vi "PhotonPoseEstimator_closestToReferencePoseStrategy.vi"(9 "ReferencePose":T2={"Translation3d"={"X"=0.0, "Y"=0.0, "Z"=0.0}, "Rotation3d"={"Q_quaternion"={"R"=1.0, "V"=[0.0, 0.0, 0.0]}}} {"Translation3d"."Z" format="%14.3f"; "Translation3d"."Y" format="%14.3f"; "Translation3d"."X" format="%14.3f"}, 10 "CameraResult":T11, 11 "PhotonPoseEstimator_REF":T1) -> (1 "Pos Found":bool, 3 "PhotonEstimatedRobotPose":T6={"EstimatedPose"={"Translation3d"={"X"=0.0, "Y"=0.0, "Z"=0.0}, "Rotation3d"={"Q_quaternion"={"R"=1.0, "V"=[0.0, 0.0, 0.0]}}}, "TimeStamp_Seconds"=0.0, "targetsUsed"=[], "Strategy"=enum."LOWEST_AMBIGUITY"} {"targetsUsed"."AltCameraToTarget"."TRANSLATION3D"."Z" format="%14.3f"; "targetsUsed"."AltCameraToTarget"."TRANSLATION3D"."Y" format="%14.3f"; "targetsUsed"."AltCameraToTarget"."TRANSLATION3D"."X" format="%14.3f"; "targetsUsed"."BestCameraToTarget"."TRANSLATION3D"."Z" format="%14.3f"; "targetsUsed"."BestCameraToTarget"."TRANSLATION3D"."Y" format="%14.3f"; "targetsUsed"."BestCameraToTarget"."TRANSLATION3D"."X" format="%14.3f"; "EstimatedPose"."Translation3d"."Z" format="%14.3f"; "EstimatedPose"."Translation3d"."Y" format="%14.3f"; "EstimatedPose"."Translation3d"."X" format="%14.3f"})   [LabVIEW 2019, in "PhotonVisionLib.lvlib"]
doc: "This is an internal function. Use Update or Update_Pipeline instead of this function.\n\nDetermine the best target based on the closest to a set Reference position"
uses:
  PhotonVisionLib.lvlib
  <vilib>/Rock Robotics/WPI/ThirdParty/JAS_Junk/TrajLib/TypeDef/QUATERNION.ctl
  <vilib>/Rock Robotics/WPI/ThirdParty/JAS_Junk/TrajLib/Trajectory_Library.lvlib
  <vilib>/Rock Robotics/WPI/ThirdParty/JAS_Junk/TrajLib/TypeDef/ROTATION3D.ctl
  <vilib>/Rock Robotics/WPI/ThirdParty/JAS_Junk/TrajLib/TypeDef/TRANSLATION3D.ctl
  <vilib>/Rock Robotics/WPI/ThirdParty/JAS_Junk/TrajLib/TypeDef/POSE3D.ctl
  TypeDef/PhotonEstimatedRobotPoseType.ctl
  Enum/PhotonPoseStrategy_ENUM.ctl
  TypeDef/TargetCornerType.ctl
  <vilib>/Rock Robotics/WPI/ThirdParty/JAS_Junk/TrajLib/TypeDef/TRANSFORM3D.ctl
  TypeDef/PhotonTrackedTargetType.ctl
  TypeDef/PhotonPipelineResultType.ctl
  <vilib>/Rock Robotics/WPI/ThirdParty/JAS_Junk/TrajLib/TypeDef/AprilTag.ctl
  <vilib>/Rock Robotics/WPI/ThirdParty/JAS_Junk/TrajLib/Enum/AprilTagFieldLayoutOrignPosition_ENUM.ctl
  <vilib>/Rock Robotics/WPI/ThirdParty/JAS_Junk/TrajLib/TypeDef/AprilTagFieldLayout.ctl
  TypeDef/PhotonPoseEstimatorType.ctl
  TypeDef/PhotonPNPResultType.ctl
  TypeDef/PhotonMultiTargetPNPResultType.ctl
  TypeDef/PhotonTargetModel.ctl
  Ref/PhotonPipelineResult_REF.ctl
  Ref/PhotonPoseEstimator_REF.ctl
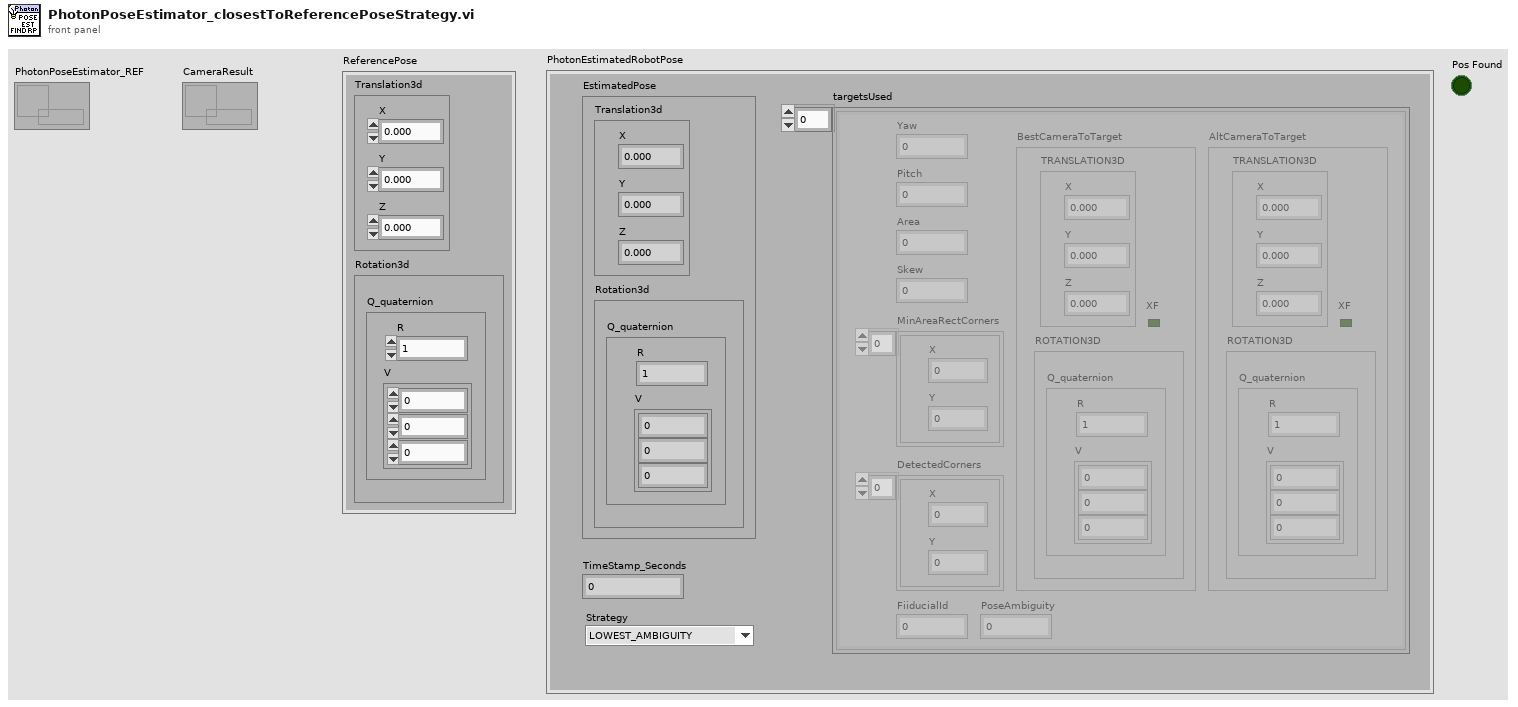
[diagram p1: front panel]
types:
  T1 = typedef "PhotonVisionLib.lvlib/PhotonPoseEstimator_REF.ctl" = refnum<data-value>
  T2 = typedef "Trajectory_Library.lvlib/POSE3D.ctl" = cluster{"Translation3d":T3, "Rotation3d":T4}
  T3 = typedef "Trajectory_Library.lvlib/TRANSLATION3D.ctl" = cluster{"X":dbl, "Y":dbl, "Z":dbl}
  T4 = typedef "Trajectory_Library.lvlib/ROTATION3D.ctl" = cluster{"Q_quaternion":T5}
  T5 = typedef "Trajectory_Library.lvlib/QUATERNION.ctl" = cluster{"R":dbl, "V":dbl[]}
  T6 = typedef "PhotonVisionLib.lvlib/PhotonEstimatedRobotPoseType.ctl" = cluster{"EstimatedPose":T2, "TimeStamp_Seconds":dbl, "targetsUsed":T7[], "Strategy":T10}
  T7 = typedef "PhotonVisionLib.lvlib/PhotonTrackedTargetType.ctl" = cluster{"Yaw":dbl, "Pitch":dbl, "Area":dbl, "Skew":dbl, "MinAreaRectCorners":T8[], "BestCameraToTarget":T9, "FiiducialId":i32, "AltCameraToTarget":T9, "PoseAmbiguity":dbl, "DetectedCorners":T8[]}
  T8 = typedef "PhotonVisionLib.lvlib/TargetCornerType.ctl" = cluster{"X":dbl, "Y":dbl}
  T9 = typedef "Trajectory_Library.lvlib/TRANSFORM3D.ctl" = cluster{"TRANSLATION3D":T3, "ROTATION3D":T4, "XF":bool}
  T10 = typedef "PhotonVisionLib.lvlib/PhotonPoseStrategy_ENUM.ctl" = enum16{"LOWEST_AMBIGUITY", "CLOSEST_TO_CAMERA_HEIGHT", "CLOSEST_TO_REFERENCE_POSE", "CLOSEST_TO_LAST_POSE", "AVERAGE_BEST_TARGETS", "MULTI_TAG_PNP_ON_COPROCESSOR", "MULTI_TAG_PNP_ON_RIO"}
  T11 = typedef "PhotonVisionLib.lvlib/PhotonPipelineResult_REF.ctl" = refnum<data-value>
  T12 = typedef "Trajectory_Library.lvlib/AprilTagFieldLayout.ctl" = cluster{"AprilTagMap":map{i32, T13}, "FieldLength":dbl, "FieldWidth":dbl, "OriginPosition ":T14, "OriginPose3d":T2}
  T13 = typedef "Trajectory_Library.lvlib/AprilTag.ctl" = cluster{"ID":i32, "POSE3D":T2}
  T14 = typedef "Trajectory_Library.lvlib/AprilTagFieldLayoutOrignPosition_ENUM.ctl" = enum16{"kBlueAllianceWallRightSide,", "kRedAllianceWallRightSide,"}
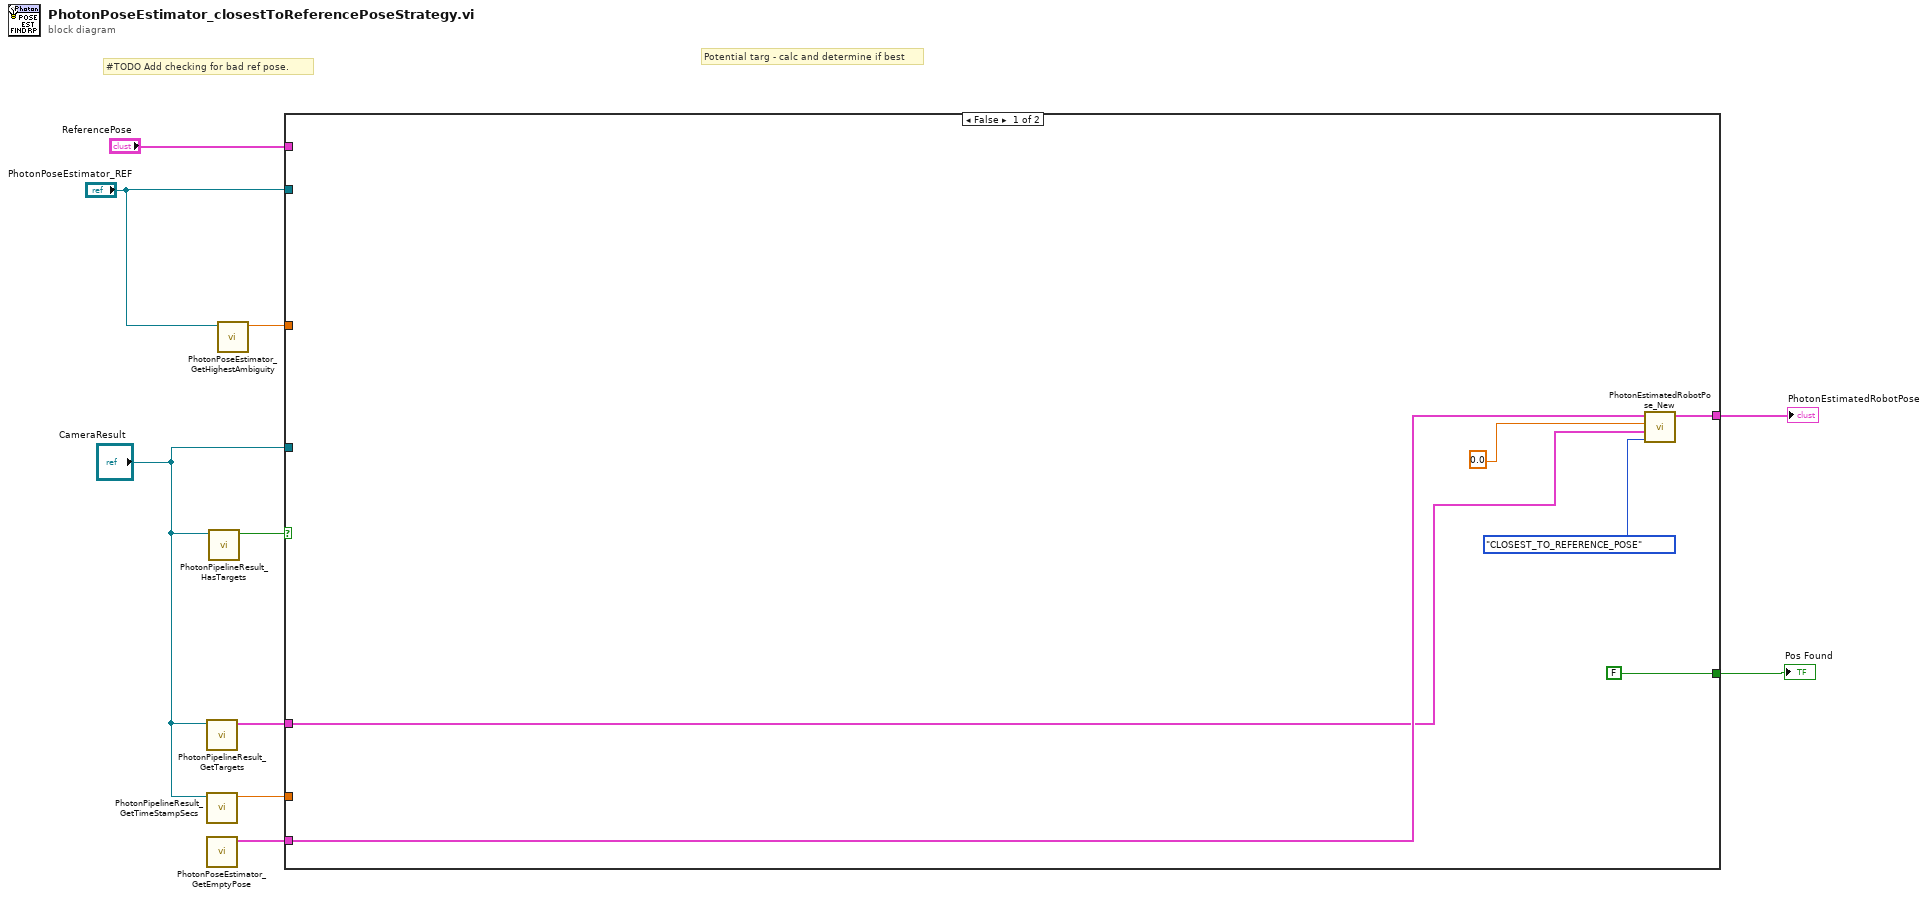
[diagram p0: block diagram]
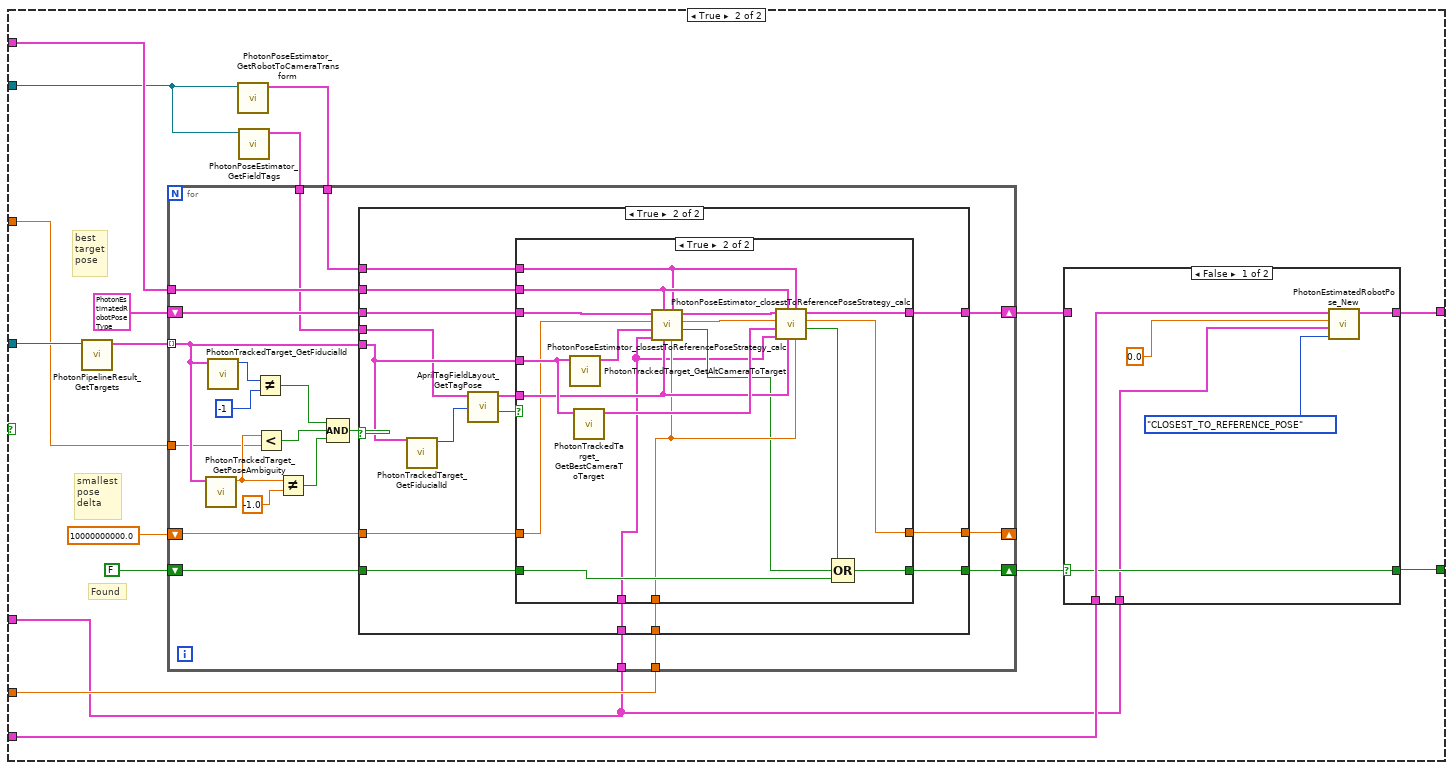
[diagram p2: hidden frame]
diagram:
  # "#TODO Add checking for bad ref pose."
  # "Potential targ - calc and determine if best"
  n1 = call "PhotonPipelineResult_GetTargets.vi"("PhotonPipelineResult_REF"="CameraResult") -> ("Targets"=w1:T7[])  [unwired: 10 in]
  n2 = call "PhotonPipelineResult_GetTimeStampSecs.vi"("PhotonPipelineResult_REF"="CameraResult") -> ("TimeStampSec"=w9:dbl)  [unwired: 10 in]
  n3 = call "PhotonPoseEstimator_GetEmptyPose.vi"() -> ("EmptyPose"=w8:T2)  [unwired: 11 in]
  n4 = call "PhotonPipelineResult_HasTargets.vi"("PhotonPipelineResult_REF"="CameraResult") -> ("HasTargets"=w10:bool)  [unwired: 10 in]
  n5 = call "PhotonPoseEstimator_GetHighestAmbiguity.vi"("PhotonPoseEstimator"="PhotonPoseEstimator_REF") -> ("HighestAmbiguity"=w3:dbl)  [unwired: 10 in]
  n6 = case shown="False" w10 {
    tunnel: "CameraResult" -> [_ w30]
    tunnel: [FALSE ("Found") w26] -> w5
    tunnel: "PhotonPoseEstimator_REF" -> [_ w19]
    tunnel: w9 -> [_ w28]
    tunnel: [w15 w24] -> w6
    tunnel: w8 -> [w14 w23]
    tunnel: "ReferencePose" -> [_ w21]
    tunnel: w3 -> [_ w22]
    tunnel: w1 -> [w11 w17]
    frame False {
      n7 = call "PhotonEstimatedRobotPose_New.vi"("Strategy"=PhotonPoseStrategy_ENUM."CLOSEST_TO_REFERENCE_POSE", "targetsUsed"=w11, "TimeStamp_Seconds"=0.0, "EstimatedPose"=w14) -> ("PhotonEstimatedRobotPose"=w15:T6)  [unwired: 7 in]
    }
    frame True {
      # "smallest\npose\ndelta"
      # "best \ntarget\npose"
      # "Found"
      n8 = call "PhotonPipelineResult_GetTargets.vi"("PhotonPipelineResult_REF"=w30) -> ("Targets"=w33:T7[])  [unwired: 10 in]
      n9 = call "PhotonPoseEstimator_GetRobotToCameraTransform.vi"("PhotonPoseEstimator"=w19) -> ("RobotToCamera"=w18:T9)  [unwired: 10 in]
      n10 = call "PhotonPoseEstimator_GetFieldTags.vi"("PhotonPoseEstimator"=w19) -> ("AprilTagFieldLayout"=w20:T12)  [unwired: 10 in]
      n11 = for {
        tunnel: w33 -> [w54] mode=indexing
        shift-right: [w58] -> w25
        shift-left: T6 {"EstimatedPose"={"Translation3d"={"X"=0.0, "Y"=0.0, "Z"=0.0}, "Rotation3d"={"Q_quaternion"={"R"=1.0, "V"=[0.0, 0.0, 0.0]}}}, "TimeStamp_Seconds"=0.0, "targetsUsed"=[], "Strategy"=enum."LOWEST_AMBIGUITY"} ("PhotonEstimatedRobotPose") -> [w57]
        shift-right: [w62] -> w27
        shift-left: FALSE -> [w59]
        shift-right: [w61] -> _
        shift-left: 10000000000.0 -> [w60]
        tunnel: w28 -> [w50]
        tunnel: w22 -> [w46]
        tunnel: w21 -> [w45]
        tunnel: w20 -> [w44]
        tunnel: w18 -> [w43]
        tunnel: w17 -> [w42]
        n12 = call "PhotonTrackedTarget_GetPoseAmbiguity.vi"("TrackedTarget"=w54) -> ("Pose Ambiguity"=w49:dbl)  [unwired: 10 in]
        n13 = call "PhotonTrackedTarget_GetFiducialId.vi"("TrackedTarget"=w54) -> ("Fiducial Id"=w56:i32)  [unwired: 10 in]
        n14 = Not Equal?(x=w56, y=-1) -> (x != y?=w48:bool)
        n15 = Less?(x=w49, y=w46) -> (x < y?=w47:bool)
        n16 = Not Equal?(x=w49, y=-1.0) -> (x != y?=w52:bool)
        n17 = Compound Arithmetic op=AND(w48, w47, w52) -> (w51:bool)
        n18 = case shown="True" w51 {
          tunnel: [w64 w73] -> w62
          tunnel: [w65 w79] -> w61
          tunnel: w60 -> [w65 w72]
          tunnel: w59 -> [w64 w71]
          tunnel: w54 -> [_ w77]
          tunnel: [w63 w78] -> w58
          tunnel: w57 -> [w63 w80]
          tunnel: w50 -> [_ w70]
          tunnel: w45 -> [_ w69]
          tunnel: w44 -> [_ w68]
          tunnel: w43 -> [_ w67]
          tunnel: w42 -> [_ w66]
          frame False {
          }
          frame True {
            n19 = call "PhotonTrackedTarget_GetFiducialId.vi"("TrackedTarget"=w77) -> ("Fiducial Id"=w76:i32)  [unwired: 10 in]
            n20 = call <vilib>:"AprilTagFieldLayout_GetTagPose.vi"("TagId"=w76, "AprilTagFieldLayout"=w68) -> ("Found"=w75:bool, "TagPose3d"=w74:T2)  [unwired: 8 in]
            n21 = case shown="True" w75 {
              tunnel: w80 -> [w83 w88]
              tunnel: [w82 w99] -> w79
              tunnel: [w83 w98] -> w78
              tunnel: w77 -> [_ w97]
              tunnel: w74 -> [_ w96]
              tunnel: [w81 w95] -> w73
              tunnel: w72 -> [w82 w87]
              tunnel: w71 -> [w81 w94]
              tunnel: w70 -> [_ w93]
              tunnel: w69 -> [_ w86]
              tunnel: w67 -> [_ w85]
              tunnel: w66 -> [_ w84]
              frame False {
              }
              frame True {
                n22 = call "PhotonTrackedTarget_GetAltCameraToTarget.vi"("TrackedTarget"=w97) -> ("AltCameraToTarget"=w100:T9)  [unwired: 9 in, 1 out]
                n23 = call "PhotonTrackedTarget_GetBestCameraToTarget.vi"("TrackedTarget"=w97) -> ("BestCameraToTarget"=w101:T9)  [unwired: 9 in, 1 out]
                n24 = call "PhotonPoseEstimator_closestToReferencePoseStrategy_calc.vi"("TimeStamp"=w93, "RobotToCamera"=w85, "FieldTargetPose"=w96, "Reference Pose"=w86, "Targets"=w84, "TransformToEvaluate"=w100, "SmallestDistToReff"=w87, "CurrentBestTrackedTarg"=w88) -> ("Found New Best"=w91:bool, "SmallestDistToRef"=w90:dbl, "PhotonEstimatedRobotPose"=w89:T6)  [unwired: 1 in]
                n25 = call "PhotonPoseEstimator_closestToReferencePoseStrategy_calc.vi"("TimeStamp"=w93, "RobotToCamera"=w85, "FieldTargetPose"=w96, "Reference Pose"=w86, "Targets"=w84, "TransformToEvaluate"=w101, "SmallestDistToReff"=w90, "CurrentBestTrackedTarg"=w89) -> ("Found New Best"=w92:bool, "SmallestDistToRef"=w99:dbl, "PhotonEstimatedRobotPose"=w98:T6)  [unwired: 1 in]
                n26 = Compound Arithmetic op=OR(w92, w91, w94) -> (w95:bool)
              }
            }
          }
        }
      }
      n27 = case shown="False" w27 {
        selector: w27 -> [w37 w41]
        tunnel: [w37 w41] -> w26
        tunnel: [w38 w40] -> w24
        tunnel: w25 -> [_ w40]
        tunnel: w23 -> [w39 _]
        tunnel: w17 -> [w34 _]
        frame False {
          n28 = call "PhotonEstimatedRobotPose_New.vi"("Strategy"=PhotonPoseStrategy_ENUM."CLOSEST_TO_REFERENCE_POSE", "targetsUsed"=w34, "TimeStamp_Seconds"=0.0, "EstimatedPose"=w39) -> ("PhotonEstimatedRobotPose"=w38:T6)  [unwired: 7 in]
        }
        frame True {
        }
      }
    }
  }
  "PhotonEstimatedRobotPose" <- w6
  "Pos Found" <- w5
